vi "oax_Check Tacho Channel Selection.vi"(8 "error in (no error)":errorcluster, 10 "Channels":T1, 11 "tachometer channel":u16(ring) items=["ch 0", "ch 1", "ch 2", "ch 3", "ch 4", "ch 5", "ch 6", "ch 7", "digital tacho"]) -> (0 "error out":errorcluster, 3 "tachometer channel out":u16(ring) items=["ch 0", "ch 1", "ch 2", "ch 3", "ch 4", "ch 5", "ch 6", "ch 7", "digital tacho"])   [LabVIEW 2017]
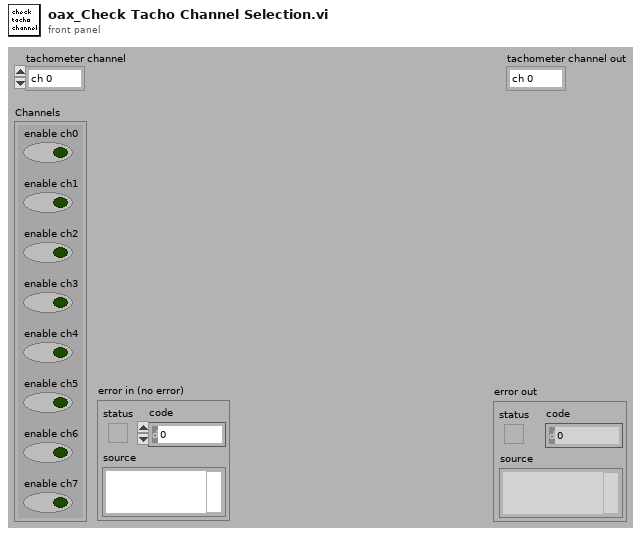
[diagram p1: front panel]
types:
  T1 = cluster{"enable ch0":bool, "enable ch1":bool, "enable ch2":bool, "enable ch3":bool, "enable ch4":bool, "enable ch5":bool, "enable ch6":bool, "enable ch7":bool}
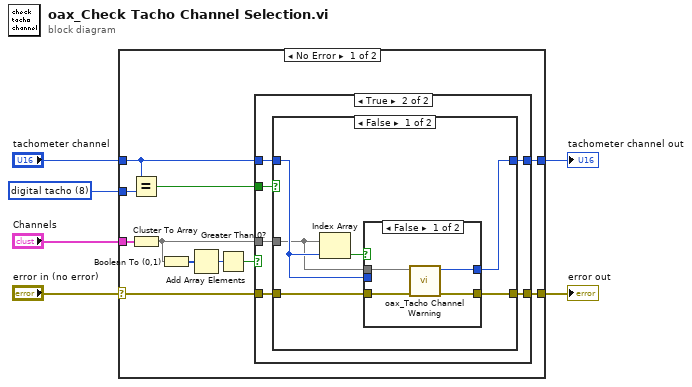
[diagram p0: block diagram]
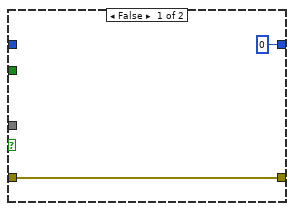
[diagram p2: hidden frame]
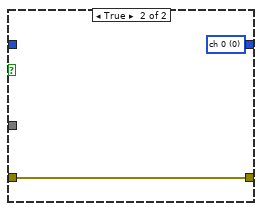
[diagram p4: hidden frame]
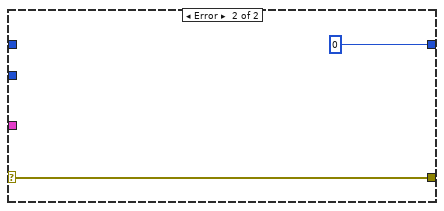
[diagram p5: hidden frame]
diagram:
  w6 = u16 8 items=["ch 0", "ch 1", "ch 2", "ch 3", "ch 4", "ch 5", "ch 6", "ch 7", "digital tacho"] ("tachometer channel")
  n1 = case shown="No Error" "error in (no error)" {
    selector: "error in (no error)" -> [w11 w41]
    tunnel: w6 -> [w17 _]
    tunnel: "Channels" -> [w16 _]
    tunnel: [w14 u16 0 ("tachometer channel")] -> w4
    tunnel: [w13 w41] -> w3
    tunnel: "tachometer channel" -> [w12 _]
    frame No Error {
      n2 = Equal?(x=w12, y=w17) -> (x = y?=w15:bool)
      n3 = Cluster To Array(cluster=w16) -> (array=w10:bool[])
      n4 = Boolean To (0,1)(Boolean=w10) -> (0, 1=w9:i16[])
      n5 = Add Array Elements(numeric array=w9) -> (sum=w8:i16)
      n6 = Greater Than 0?(x=w8) -> (x > 0?=w7:bool)
      n7 = case shown="True" w7 {
        tunnel: w15 -> [_ w25]
        tunnel: [u16 0 ("tachometer channel") w24] -> w14
        tunnel: [w19 w23] -> w13
        tunnel: w12 -> [_ w22]
        tunnel: w11 -> [w19 w21]
        tunnel: w10 -> [_ w20]
        frame False {
        }
        frame True {
          n8 = case shown="False" w25 {
            tunnel: [w28 w39] -> w24
            tunnel: w21 -> [w30 w38]
            tunnel: [w29 w38] -> w23
            tunnel: w20 -> [w26 _]
            tunnel: w22 -> [w27 _]
            frame False {
              n9 = Index Array(array=w26, index=w27) -> (element=w31:bool)
              n10 = case shown="False" w31 {
                tunnel: w30 -> [w33 w37]
                tunnel: [w32 w37] -> w29
                tunnel: [w35 w36] -> w28
                tunnel: w27 -> [_ w36]
                tunnel: w26 -> [w34 _]
                frame False {
                  n11 = call <vilib>:"oax_Tacho Channel Warning.vi"("error in (no error)"=w33, "Channels"=w34) -> ("error out"=w32:errorcluster, "tachometer channel 2"=w35:u16)  [unwired: 8 in]
                }
                frame True {
                }
              }
            }
            frame True {
              w39 = u16 0 items=["ch 0", "ch 1", "ch 2", "ch 3", "ch 4", "ch 5", "ch 6", "ch 7", "digital tacho"] ("tachometer channel")
            }
          }
        }
      }
    }
    frame Error {
    }
  }
  "error out" <- w3
  "tachometer channel out" <- w4
